vi "OptimizationFunction.vi"(9 "output selector":T1, 10 "data":variant, 11 "Input parameters":dbl[](array[numeric])=[8.0, -2.0, 0.02] step=1e-10 format="%#.8f") -> (0 "error out":errorcluster, 1 "Inequality Constraints":dbl[](array[numeric]), 2 "Equality Constraints":dbl[](array[numeric]), 3 "Objective Functions":dbl[](array[numeric]))   [LabVIEW 2020]
uses:
  <vilib>/gmath/NumericalOptimization/cno_output select.ctl
  <vilib>/gmath/NI_Gmath.lvlib
panel:
  in  "X":dbl[](array[numeric])
  in  "Goal function":dbl[](array[numeric])=[-0.407, 0.781, 0.00845, -0.0056] step=1e-10 format="%#.8f"
  out "Measured":waveform(dbl)(graph)={"t0"=timestamp(0 s since 1904-01-01), "dt"=1.0, "Y"=array[3075 elements]}
  out "error":waveform(dbl)(graph)={"t0"=timestamp(0 s since 1904-01-01), "dt"=1.0, "Y"=array[3075 elements]}
  # "A*t^3+B*t^2+C*t+D"
  # "D"
  # "C"
  # "B"
  # "A"
  # "D"
  # "C"
  # "A*t^3+B*t^2+C*t+D"
  # "B"
  # "A"
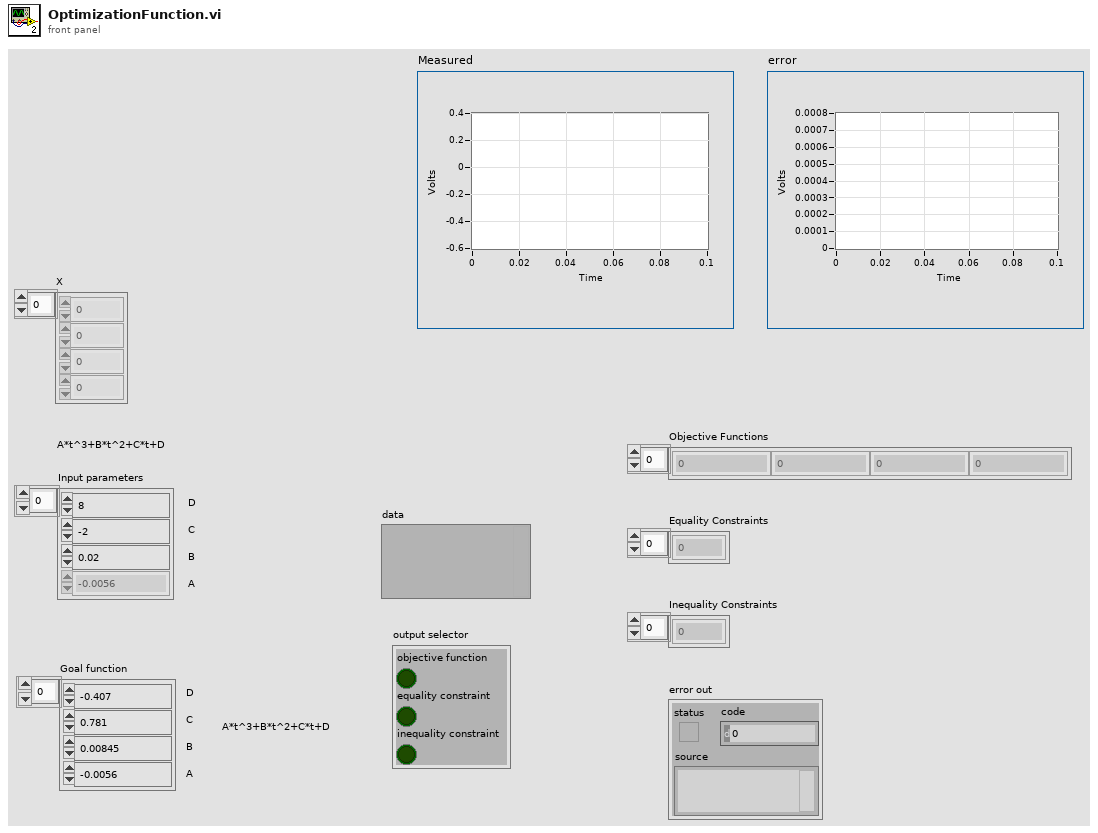
[diagram p1: front panel]
types:
  T1 = typedef "NI_Gmath.lvlib/cno_output select.ctl" = cluster{"objective function":bool, "equality constraint":bool, "inequality constraint":bool}
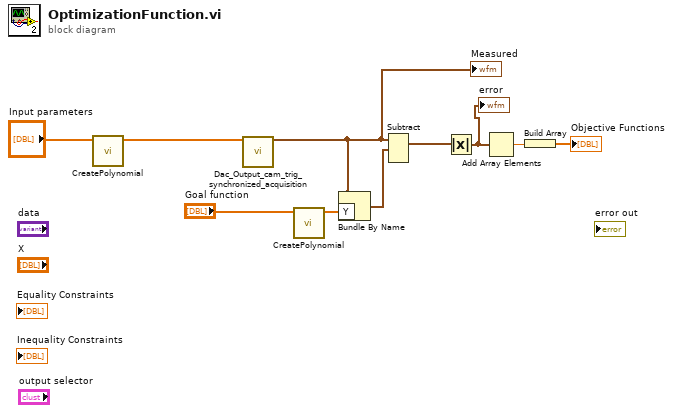
[diagram p0: block diagram]
diagram:
  n1 = call "CreatePolynomial.vi"("P(x)"="Input parameters") -> ("Waveform Graph"=w5:dbl[])  [unwired: 9 in]
  n2 = call "Dac_Output_cam_trig_synchronized_acquisition.vi"("LabVIEW generated Sawtooth input"=w5) -> ("Measured voltage"=w6:waveform(dbl))  [unwired: 18 in]
  "Measured" <- w6
  n3 = call "CreatePolynomial.vi"("P(x)"="Goal function") -> ("Waveform Graph"=w4:dbl[])  [unwired: 9 in]
  n4 = Bundle By Name(cluster=w6, "Y"=w4) -> (w7:waveform(dbl))
  n5 = Subtract(1:w7, 2:w6) -> (0:w9:waveform(dbl))  [unwired: 1 in, 1 out]
  n6 = Absolute Value(x=w9) -> (abs(x)=w8:waveform(dbl))
  "error" <- w8
  n7 = Add Array Elements(numeric array=w8) -> (sum=w2:dbl)
  n8 = Build Array(w2) -> (→"Objective Functions":dbl[])
